vi "Open Spreadsheet File (Consecutive Delimeters).vi"(8 "error in (no error)":errorcluster, 10 "delimiters (\\s)":string[](array[string])=[" "], 11 "File":path caption="Spreadsheet File") -> (0 "error out":errorcluster, 3 "Array":string[][](array[string]))   [LabVIEW 2010]
uses:
  <vilib>/Utility/file.llb/Read From Spreadsheet File (string).vi
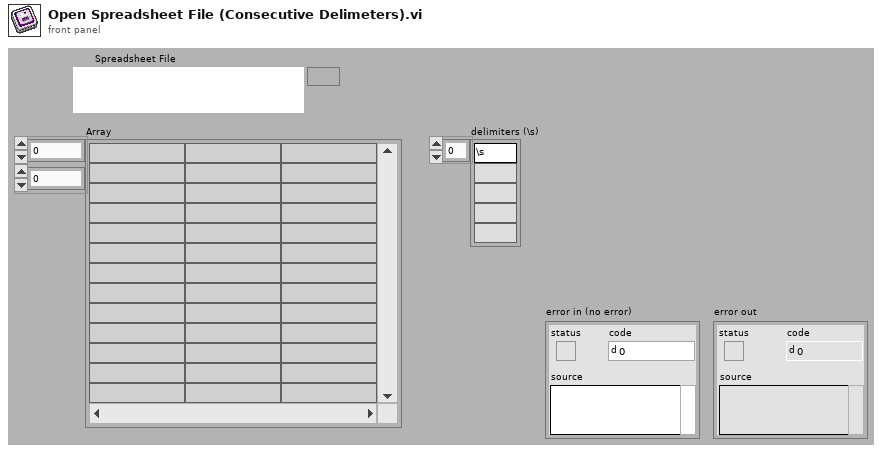
[diagram p1: front panel]
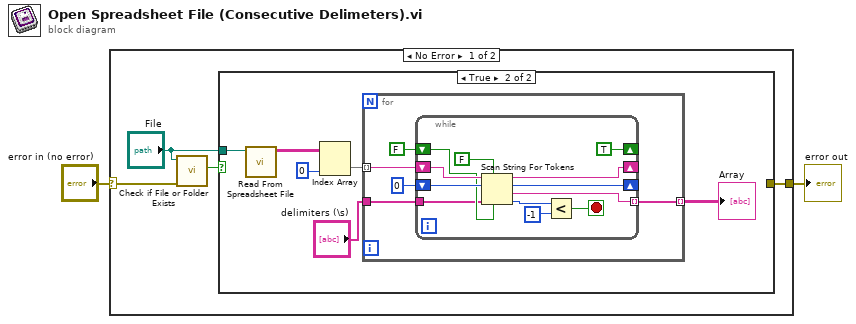
[diagram p0: block diagram]
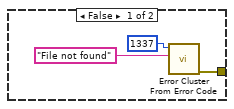
[diagram p2: hidden frame]
diagram:
  n1 = case shown="No Error" "error in (no error)" {
    selector: "error in (no error)" -> [w4 w33]
    tunnel: [w3 w33] -> w1
    frame No Error {
      n2 = call <vilib>:"Check if File or Folder Exists.vi"("error in (no error)"=w4, "path"="File") -> ("file or folder exists?"=w5:bool)  [unwired: 7 in, 2 out]
      n3 = case shown="True" w5 {
        tunnel: "File" -> [_ w10]
        tunnel: [w9 _] -> w3
        frame False {
          n4 = call <vilib>:"Error Cluster From Error Code.vi"("error message (\"\")"="File not found" ("error message (\"\")"), "error code (0)"=1337) -> ("error out"=w9:errorcluster)  [unwired: 7 in]
        }
        frame True {
          n5 = call-poly <vilib>:"Read From Spreadsheet File.vi"("file path (dialog if empty)"=w10) -> ("all rows"=w13:string[][])  [unwired: 6 in, 4 out]
          n6 = Index Array(array=w13, index (col)=0 ("disabled index (col)")) -> (element=w14:string[])  [unwired: 1 in]
          n7 = for {
            tunnel: w14 -> [w20] mode=indexing
            tunnel: [w19] -> w12 mode=indexing
            tunnel: "delimiters (\\s)" -> [w16]
            n8 = while {
              shift-right: [w30] -> _
              shift-left: w20 -> [w31]
              tunnel: [w29] -> w19 mode=indexing
              shift-right: [w28] -> _
              shift-left: 0 ("offset past token") -> [w27]
              shift-right: [TRUE ("allow empty tokens? (F)")] -> _
              shift-left: FALSE ("allow empty tokens? (F)") -> [w23]
              tunnel: w16 -> [w21]
              stop <- w24 stop-if-true
              n9 = Scan String For Tokens(4:w23, 5:FALSE ("allow empty tokens? (F)"), 6:w21, 8:w27, 9:w31) -> (0:w26:i32, 1:w29:string, 2:w28:i32, 3:w30:string)  [unwired: 1 in]
              n10 = Less?(x=w26, y=-1) -> (x < y?=w24:bool)
            }
          }
          "Array" <- w12
        }
      }
    }
    frame Error {
    }
  }
  "error out" <- w1
